vi "Do.vi"(8 "error in (no error)":errorcluster, 10 "Actor in":refnum<class "Actor.lvclass">, 11 "Load Image from File Msg":refnum<class "Load Image from File Msg.lvclass">) -> (0 "error out":errorcluster, 2 "Actor out":refnum<class "Actor.lvclass">)   [LabVIEW 2014, in "HIJ Vision File Viewer.lvlib" / "Load Image from File Msg.lvclass"]
doc: "This VI delivers the message to the actor by calling the appropriate method(s) on the actor."
uses:
  Load Image from File Msg.lvclass
  <vilib>/ActorFramework/Actor/Actor.lvclass
  HIJ Vision File Viewer/HIJ Vision File Viewer.lvclass
  Load Image from File Msg.lvclass/Load Image from File Msg.ctl
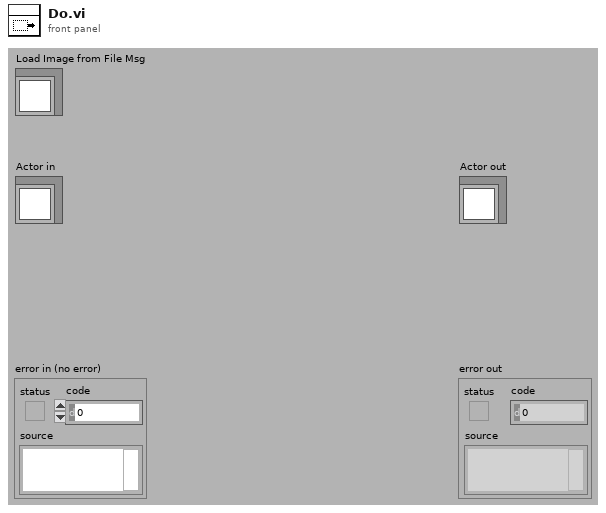
[diagram p1: front panel]
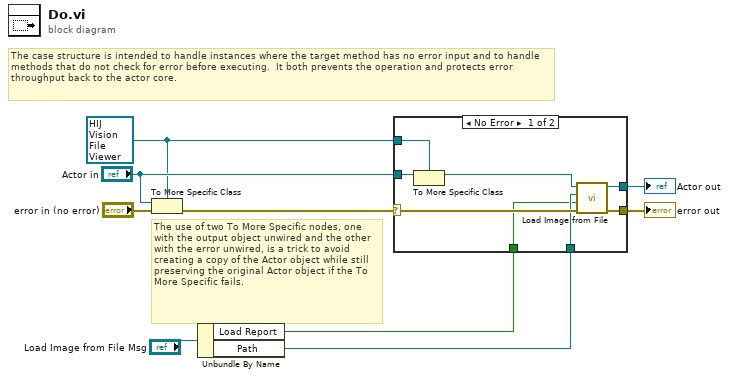
[diagram p0: block diagram]
diagram:
  w4 = refnum<class "HIJ Vision File Viewer.lvclass"> refnum ("Actor in")
  # "The use of two To More Specific nodes, one with the output object unwired and the other with the error unwired, is a trick to avoid creating a copy of the Actor object while still preserving the original Actor object if the To More Specific fails."
  # "The case structure is intended to handle instances where the target method has no error input and to handle methods that do not check for error before executing.  It both prevents the operation and protects error throughput back to the actor core."
  n1 = To More Specific Class(target class=w4, reference="Actor in", error in="error in (no error)") -> (error out=w8:errorcluster)  [unwired: 1 out]
  n2 = Unbundle By Name("Load Image from File Msg") -> ("Load Report"=w1:bool, "Path"=w2:path)
  n3 = case shown="No Error" w8 {
    selector: w8 -> [w15 w19]
    tunnel: [w17 w19] -> w7
    tunnel: [w16 w18] -> w6
    tunnel: "Actor in" -> [w14 w18]
    tunnel: w4 -> [w13 _]
    tunnel: w2 -> [w11 _]
    tunnel: w1 -> [w10 _]
    frame No Error {
      n4 = To More Specific Class(target class=w13, reference=w14) -> (specific class reference=w12:refnum<class "HIJ Vision File Viewer.lvclass">)  [unwired: 1 in, 1 out]
      n5 = call-dynamic "Load Image from File.vi"("error in (no error)"=w15, "Load Report"=w10, "Image"=w11, "HIJ Vision File Viewer in"=w12) -> ("error out"=w17:errorcluster, "HIJ Vision File Viewer out"=w16:refnum<class "HIJ Vision File Viewer.lvclass">)  [unwired: 6 in]
    }
    frame Error {
      # "If type check fails, pass the original object out again."
    }
  }
  "error out" <- w7
  "Actor out" <- w6
